vi "Config_INTAN (SubVI).vi"(1 "Mode":string, 2 "Channel":string, 3 "Frequency Band Width":string, 4 "Intan":u16) -> (0 "String":string)   [LabVIEW 2018]
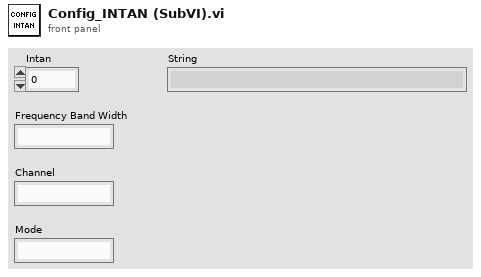
[diagram p1: front panel]
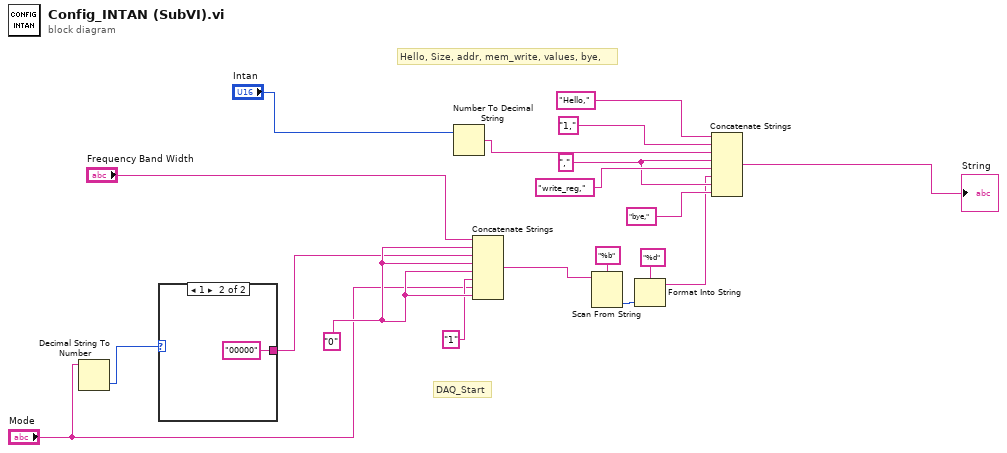
[diagram p0: block diagram]
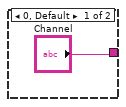
[diagram p2: hidden frame]
diagram:
  w13 = "," ("string")
  w5 = "0"
  # "DAQ_Start"
  # "Hello, Size, addr, mem_write, values, bye,"
  n1 = Decimal String To Number(string="Mode") -> (number=w2:i32)  [unwired: 2 in, 1 out]
  n2 = case shown="1" w2 {
    tunnel: ["Channel" "00000" ("Channel")] -> w1
    frame 0, Default {
    }
    frame 1 {
    }
  }
  n3 = Number To Decimal String(number="Intan") -> (decimal integer string=w15:string)  [unwired: 1 in]
  n4 = Concatenate Strings("Frequency Band Width", w5, w1, w5, w5, "1" ("string"), "Mode", w5) -> (w10:string)
  n5 = Scan From String(format string="%b", input string=w10) -> (output 1=w8:i32)  [unwired: 3 in, 3 out]
  n6 = Format Into String(format string="%d", w8) -> (resulting string=w6:string)  [unwired: 2 in, 1 out]
  n7 = Concatenate Strings("Hello," ("string"), "1," ("string"), w15, w13, "write_reg," ("string"), w6, w13, "bye," ("string")) -> (→"String":string)
